vi "Get a raw Channel Data (input for Analyser).vi"() -> (0 "Data Output":T2 {"Data Channels" format="%.2f"})   [LabVIEW 2013]
panel:
  in  "Tab Control":enum32{"Channels", "Defaults"}(tab)
  in  "Additional Channels":T1(array[cluster])=[{"Channel No."=10, "Scaling Factor"=1.0, "Channel Name"=0, "Offset Factor"=0}, {"Channel No."=15, "Scaling Factor"=1.0, "Channel Name"=1, "Offset Factor"=0}] {"Channel Name" items=["Vertical Eye", "Stimulus"]; "Scaling Factor" format="%.4e"}
  in  "Available Channel Names":string[](array[string])=["Vertical Eye", "Stimulus"]
  # "Copyright Americo A. Migliaccio (c) 2002 All Rights Reserved by Author"
  # "Channel          Offset            Gain"
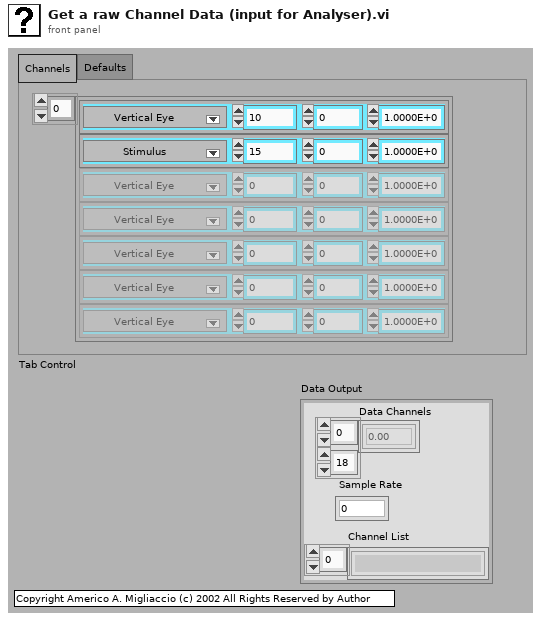
[diagram p1: front panel]
types:
  T1 = cluster{"Channel No.":i32, "Scaling Factor":dbl, "Channel Name":u16, "Offset Factor":i32}[]
  T2 = cluster{"Data Channels":dbl[][], "Sample Rate":i32, "Channel List":string[]}
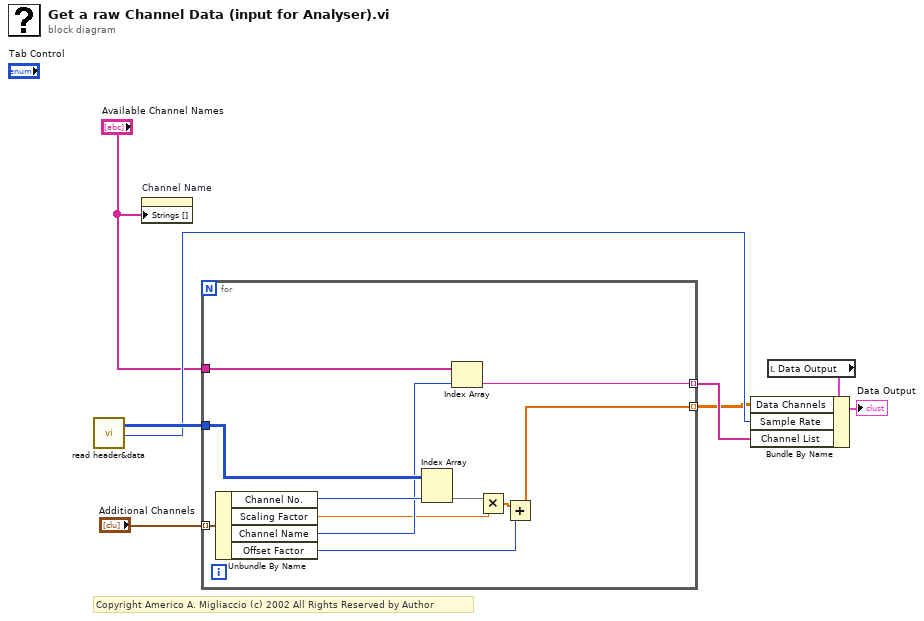
[diagram p0: block diagram]
diagram:
  # "Copyright Americo A. Migliaccio (c) 2002 All Rights Reserved by Author"
  n1 = call "read header&data.vi"() -> ("ADD1"=w4:i32, "Data Array"=w8:i16[][])  [unwired: 4 in, 14 out]
  n2 = property on="Channel Name" class="Ring (strict)"("Strings []"="Available Channel Names") -> ()  [unwired: 2 in, 2 out]
  n3 = for {
    tunnel: w8 -> [w19]
    tunnel: "Additional Channels" -> [w18] mode=indexing
    tunnel: "Available Channel Names" -> [w16]
    tunnel: [w14] -> w2 mode=indexing
    tunnel: [w9] -> w1 mode=indexing
    n4 = Unbundle By Name(w18) -> ("Channel No."=w17:i32, "Scaling Factor"=w12:dbl, "Channel Name"=w15:u16, "Offset Factor"=w10:i32)
    n5 = Index Array(array=w19, index (col)=w17) -> (element=w13:i16[])  [unwired: 1 in]
    n6 = Index Array(array=w16, index=w15) -> (element=w14:string)
    n7 = Multiply(x=w13, y=w12) -> (x*y=w11:dbl[])
    n8 = Add(x=w11, y=w10) -> (x+y=w9:dbl[])
  }
  n9 = local read "Data Output"() -> (w5:T2)
  n10 = Bundle By Name(cluster=w5, "Data Channels"=w1, "Sample Rate"=w4, "Channel List"=w2) -> (→"Data Output":T2)
